vi "3.1.1_ECO_Power_Tune.vi"(6 "Data in":T1, 8 "error in (no error)":errorcluster, 9 "AllControls In":T2, 10 "?":T3, 11 "Message Queue out":T4) -> (0 "error out":errorcluster, 1 "Flow":string, 2 "Data":T3, 3 "Message Queue Out":T4, 4 "Data out":T1)   [LabVIEW 2017]
uses:
  Depends/AMC/subVIs/TypeDefs/amc_Message Queue.ctl
  Depends/AMC/subVIs/TypeDefs/amc_Message.ctl
  Depends/Tools/Keyed Array/Tools_KeyedArray KeyedArray.ctl
  Ctrls/Data.ctl
  Ctrls/CSV_Data.ctl
  Ctrls/AllControls.ctl
  DIPC 692 Daemon API/typdef/get_parameter.ctl
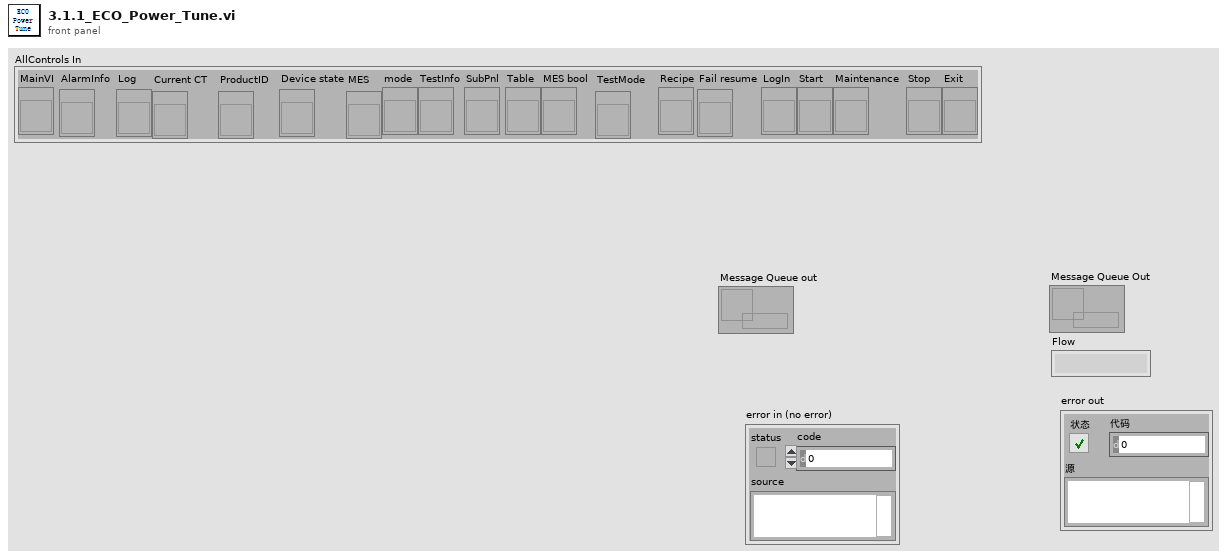
[diagram p1: front panel]
types:
  T1 = typedef "CSV_Data.ctl" = cluster{"Initialisation":cluster{"LMT - Connect UUT (con COM)":string, "LMT - Software Version (rrel)":string, "LMT - Write SKU file (wskuc)":string, "LMT - SKU file name":string, "Connect UUT DDM":string, "Read DDM EOL Timestamp - Mode":string, "Read DDM EOL Timestamp - Timestamp":string, "Read DDM EOL Timestamp - Rig ID":string, "Read DDM EOL Timestamp - Passmark ID":string, "Read DDM EOL Timestamp - Passmark Rev":string, "Software Version before flashing":string, "Read Hardware Serial":string, "UUT DDM SN":string, "Compare DDM SN with MES SN":string, "Backup PCBA Calibration EEPROM Response - CAL":string, "Flash Firmware Version":string, "Check SW Version":string, "Read DDM SW Version after flashing":string, "Set SKU Config":string, "Ready Status":string, "Set Device Mode to EOL":string, "DDM Parameter - Voltage":string, "DDM Parameter - Current":string, "DDM Parameter - Power":string, "DDM Parameter - Speed":string, "DDM Parameter - Pressure":string, "Tester Parameter - Voltage":string, "Tester Parameter - Current":string, "Tester Parameter - Power":string, "Tester Parameter - Ambient Pressure":string, "Tester Parameter - Ambient Temperature":string, "Calculated Parameter - DDM Pressure Corrected":string, "Calculated Parameter - DDM Real Power":string, "Calculated Parameter - Delta V":string}, "BEMF_Calibration":cluster{"Calibration Result - eol_cold_bemf_temp":string, "DDM Ambient Temp":string, "Restriction Plate Diameter":string, "Calibration Result - eol_bemf_mp_cold_coef_a":string, "Calibration Result - eol_bemf_mp_cold_coef_b":string, "Calibration Result - eol_bemf_mp_cold_coef_c":string, "Calibration Result - eol_bemf_lsi_cold_ref_coeffs":string, "Get - Calibration Result - eol_bemf_lsi_speed":string, "Get - Calibration Result - eol_bemf_lsi_integral_0":string, "Calibration Result - eol_bemf_lsi_integral_1":string, "Get - Calibration Result - eol_bemf_lsi_integral_2":string, "Get - Calibration Result - eol_cold_bemf":string, "Get - Calibration Result - eol_cold_bemf_fisf":string, "Finalise Calibration":string, "Compare -Calibration Result - eol_cold_bemf":string, "Compare -Calibration Result - eol_cold_bemf_fisf":string}, "ECO":cluster{"Reset Power Tune":string, "Reset BEMF FISF Calibration":string, "Restriction Plate Diameter":string, "ECO - Stabilisation Time":string, "ECO - DDM Parameter - Voltage":string, "ECO - DDM Parameter - Current":string, "ECO - DDM Parameter - Power":string, "ECO - DDM Parameter - Measured Power":string, "ECO - DDM Parameter - Speed":string, "ECO - DDM Parameter - Pressure":string, "ECO - Tester Parameter - Voltage":string, "ECO - Tester Parameter - Current":string, "ECO - Tester Parameter - Power":string, "ECO - Tester Parameter - Ambient Pressure":string, "ECO - Tester Parameter - Ambient Temperature":string, "ECO - Tester Parameter - Ambient Humidity":string, "ECO - Calculated Parameter - DDM Pressure Corrected":string, "ECO - Calculated Parameter - DDM Real Power":string, "ECO - Calculated Parameter - Delta V":string, "ECO - Calculated Parameter - Flowrate":string, "ECO - Calculated Parameter - Airwatt":string, "ECO - Formula":string, "PT ECO - Power Tune Mode Status":string}, "BOOST":cluster{"Restriction Plate Diameter":string, "BOOST - Stabilisation Time":string, "BOOST - DDM Parameter - Voltage":string, "BOOST - DDM Parameter - Current":string, "BOOST - DDM Parameter - Power":string, "BOOST - DDM Parameter - Measured Power":string, "BOOST - DDM Parameter - Speed":string, "BOOST - DDM Parameter - Pressure":string, "BOOST - Tester Parameter - Voltage":string, "BOOST - Tester Parameter - Current":string, "BOOST - Tester Parameter - Power":string, "BOOST - Tester Parameter - Ambient Pressure":string, "BOOST - Tester Parameter - Ambient Temperature":string, "BOOST - Tester Parameter - Ambient Humidity":string, "BOOST - Calculated Parameter - DDM Pressure Corrected":string, "BOOST - Calculated Parameter - DDM Real Power":string, "BOOST - Calculated Parameter - Delta V":string, "BOOST - Calculated Parameter - Flowrate":string, "BOOST - Calculated Parameter - Airwatt":string, "BOOST - Get AM Presence":string, "Air Muscle Turn Off Status":string, "BOOST - Air Muscle Calculated Parameter - Airwatt B":string, "BOOST - Air Muscle Calculate Airwatt Delta":string, "PT BOOST - Power Tune Mode Status":string, "Finalise Calibration":string, "ECO - Get AW Calibration value":string, "BOOST - Get AW Calibration value":string}, "MAX":cluster{"Restriction Plate Diameter":string, "MAX - Stabilisation Time":string, "Get Average Delta Tmag (LSIdelta_FISFdelta_LSItmag_FISFtmag_IIRtmag)":string, "Get Average Delta Tmag FISF":string, "MAX - DDM Parameter - Voltage":string, "MAX - DDM Parameter - Current":string, "MAX - DDM Parameter - Power":string, "MAX - DDM Parameter - Measured Power":string, "MAX - DDM Parameter - Speed":string, "MAX - DDM Parameter - Pressure":string, "MAX - Tester Parameter - Voltage":string, "MAX - Tester Parameter - Current":string, "MAX - Tester Parameter - Power":string, "MAX - Tester Parameter - Ambient Pressure":string, "MAX - Tester Parameter - Ambient Temperature":string, "MAX - Tester Parameter - Ambient Humidity":string, "MAX - Calculated Parameter - DDM Pressure Corrected":string, "MAX - Calculated Parameter - DDM Real Power":string, "MAX - Calculated Parameter - Delta V":string, "MAX - Calculated Parameter - Flowrate":string, "MAX - Calculated Parameter - Airwatt":string, "MAX_FISF_Check_Average_Delta_Tmag":string, "MAX - FISF - BEMF Finetune Result":string, "MAX tune - Delta P1":string, "MAX tune - Calculated Parameter - Airwatt":string, "Calculate Delta Airwatts - MAX finetune - Delta P2":string, "MAX finetune - DDM Parameter - Voltage":string, "MAX finetune - DDM Parameter - Current":string, "MAX finetune - DDM Parameter - Power":string, "MAX finetune - DDM Parameter - Measured Power":string, "MAX finetune - DDM Parameter - Speed":string, "MAX finetune - DDM Parameter - Pressure":string, "MAX finetune - Tester Parameter - Voltage":string, "MAX finetune - Tester Parameter - Current":string, "MAX finetune - Tester Parameter - Power":string, "MAX finetune - Tester Parameter - Ambient Pressure":string, "MAX finetune - Tester Parameter - Ambient Temperature":string, "MAX finetune - Tester Parameter - Ambient Humidity":string, "MAX finetune - Calculated Parameter - DDM Pressure Corrected":string, "MAX finetune - Calculated Parameter - DDM Real Power":string, "MAX finetune - Calculated Parameter - Delta V":string, "MAX finetune - Calculated Parameter - Flowrate":string, "MAX finetune - Calculated Parameter - Airwatt":string, "Check Derate Result":string, "Delta Tmag FISF":string, "Get Hot BEMF Result":string, "Calculate delta Pressure":string, "Finalise Calibration":string, "Calculate & Check Delta BEMF":string, "Delta P Airwatts Value":string}, "LL":cluster{"DDM Ambient Temp":string, "Restriction Plate Diameter":string, "LL - DDM Parameter - Voltage":string, "LL - DDM Parameter - Current":string, "LL - DDM Parameter - Power":string, "LL - DDM Parameter - Measured Power":string, "LL - DDM Parameter - Speed":string, "LL - DDM Parameter - Pressure":string, "LL - Tester Parameter - Voltage":string, "LL - Tester Parameter - Current":string, "LL - Tester Parameter - Power":string, "LL - DDM Real Power":string, "LL - Calibrate Task Detect LL":string}, "HL":cluster{"HL - DDM Parameter - Voltage":string, "HL - DDM Parameter - Current":string, "HL - DDM Parameter - Power":string, "HL - DDM Parameter - Measured Power":string, "HL - DDM Parameter - Speed":string, "HL - DDM Parameter - Pressure":string, "HL - Tester Parameter - Voltage":string, "HL - Tester Parameter - Current":string, "HL - Tester Parameter - Power":string, "HL - DDM Real Power":string, "HL - Calibrate Task Detect HL":string}, "LH":cluster{"Restriction Plate Diameter":string, "LH - DDM Parameter - Voltage":string, "LH - DDM Parameter - Current":string, "LH - DDM Parameter - Power":string, "LH - DDM Parameter - Measured Power":string, "LH - DDM Parameter - Speed":string, "LH - DDM Parameter - Pressure":string, "LH - Tester Parameter - Voltage":string, "LH - Tester Parameter - Current":string, "LH - Tester Parameter - Power":string, "LH - DDM Real Power":string, "LH - Calibrate Task Detect LH":string}, "HH":cluster{"HH - DDM Parameter - Voltage":string, "HH - DDM Parameter - Current":string, "HH - DDM Parameter - Power":string, "HH - DDM Parameter - Measured Power":string, "HH - DDM Parameter - Speed":string, "HH - DDM Parameter - Pressure":string, "HH - Tester Parameter - Voltage":string, "HH - Tester Parameter - Current":string, "HH - Tester Parameter - Power":string, "HH - DDM Real Power":string, "HH - Calibrate Task Detect HH":string}, "Inlet Blockage Calibration":cluster{"Inlet Blockage Calibration - DDM Parameter - Voltage":string, "Inlet Blockage Calibration - DDM Parameter - Current":string, "Inlet Blockage Calibration - DDM Parameter - Power":string, "Inlet Blockage Calibration - DDM Parameter - Measured Power":string, "Inlet Blockage Calibration - DDM Parameter - Speed":string, "Inlet Blockage Calibration - DDM Parameter - Pressure":string, "Inlet Blockage Calibration - Tester Parameter - Voltage":string, "Inlet Blockage Calibration - Tester Parameter - Current":string, "Inlet Blockage Calibration - Tester Parameter - Power":string, "Inlet Blockage Calibration - DDM Real Power":string, "Calibration Inlet Blockage_E":string, "Finalise Calibration":string, "Get Task Detect LL":string, "Get Task Detect HL":string, "Get Task Detect LH":string, "Get Task Detect HH":string, "Calibration Inlet Blockage":string, "Calibration eol cold bemf temp":string}, "GOOD":cluster{"GOOD UNIT - Clear EEPROM Error Log":string, "GOOD UNIT - Write Product Timestamp - Mode":string, "GOOD UNIT - Write Product Timestamp - Timestamp":string, "GOOD UNIT - Write Product Timestamp - Rig ID":string, "GOOD UNIT - Write Product Timestamp - Passmark ID":string, "GOOD UNIT - Write Product Timestamp - Passmark Rev":string, "GOOD UNIT - Set Device Mode to PROD":string, "GOOD UNIT - Backup PCBA Calibration EEPROM Response":string, "GOOD UNIT - Check Security Bit":string, "GOOD UNIT - Set Calibration Lock":string, "GOOD UNIT - Get_Calibration_Lock":string, "GOOD UNIT - Disconnect UUT":string}, "NG":cluster{"NG UNIT - Read NVM Error":string, "NG UNIT - Set Device Mode to FCT":string, "NG UNIT - Backup PCBA Calibration EEPROM Response - CAL":string, "NG UNIT - Backup PCBA Calibration EEPROM Response - ERROR":string, "NG UNIT - Backup PCBA Calibration EEPROM Response - USAGE":string, "NG UNIT - Disconnect UUT":string}, "SN":string, "Table":string[][], "Count":cluster{"Total":i32, "OK":i32, "NG":i32, "Yield":dbl}, "Start Time":timestamp, "daemon reference":refnum<k5>, "CT":dbl, "Config":string[][], "OK/NG":bool, "Station ID":string, "MES DDM SN":string, "MES PCBA SN":string, "Retest":string, "Lux":string, "Initialisation_Status":cluster{"LMT - Connect UUT (con COM)":string, "LMT - Software Version (rrel)":string, "LMT - Write SKU file (wskuc)":string, "LMT - SKU file name":string, "Connect UUT DDM":string, "Read DDM EOL Timestamp - Mode":string, "Read DDM EOL Timestamp - Timestamp":string, "Read DDM EOL Timestamp - Rig ID":string, "Read DDM EOL Timestamp - Passmark ID":string, "Read DDM EOL Timestamp - Passmark Rev":string, "Software Version before flashing":string, "Read Hardware Serial":string, "UUT DDM SN":string, "Compare DDM SN with MES SN":string, "Backup PCBA Calibration EEPROM Response - CAL":string, "Flash Firmware Version":string, "Check SW Version":string, "Read DDM SW Version after flashing":string, "Set SKU Config":string, "Ready Status":string, "Set Device Mode to EOL":string, "DDM Parameter - Voltage":string, "DDM Parameter - Current":string, "DDM Parameter - Power":string, "DDM Parameter - Speed":string, "DDM Parameter - Pressure":string, "Tester Parameter - Voltage":string, "Tester Parameter - Current":string, "Tester Parameter - Power":string, "Tester Parameter - Ambient Pressure":string, "Tester Parameter - Ambient Temperature":string, "Calculated Parameter - DDM Pressure Corrected":string, "Calculated Parameter - DDM Real Power":string, "Calculated Parameter - Delta V":string}, "BEMF_Calibration_Status":cluster{"Calibration Result - eol_cold_bemf_temp":string, "DDM Ambient Temp":string, "Restriction Plate Diameter":string, "Calibration Result - eol_bemf_mp_cold_coef_a":string, "Calibration Result - eol_bemf_mp_cold_coef_b":string, "Calibration Result - eol_bemf_mp_cold_coef_c":string, "Calibration Result - eol_bemf_lsi_cold_ref_coeffs":string, "Get - Calibration Result - eol_bemf_lsi_speed":string, "Get - Calibration Result - eol_bemf_lsi_integral_0":string, "Calibration Result - eol_bemf_lsi_integral_1":string, "Get - Calibration Result - eol_bemf_lsi_integral_2":string, "Get - Calibration Result - eol_cold_bemf":string, "Get - Calibration Result - eol_cold_bemf_fisf":string, "Finalise Calibration":string, "Compare -Calibration Result - eol_cold_bemf":string, "Compare -Calibration Result - eol_cold_bemf_fisf":string}, "ECO_Status":cluster{"Reset Power Tune":string, "Reset BEMF FISF Calibration":string, "Restriction Plate Diameter":string, "ECO - Stabilisation Time":string, "ECO - DDM Parameter - Voltage":string, "ECO - DDM Parameter - Current":string, "ECO - DDM Parameter - Power":string, "ECO - DDM Parameter - Measured Power":string, "ECO - DDM Parameter - Speed":string, "ECO - DDM Parameter - Pressure":string, "ECO - Tester Parameter - Voltage":string, "ECO - Tester Parameter - Current":string, "ECO - Tester Parameter - Power":string, "ECO - Tester Parameter - Ambient Pressure":string, "ECO - Tester Parameter - Ambient Temperature":string, "ECO - Tester Parameter - Ambient Humidity":string, "ECO - Calculated Parameter - DDM Pressure Corrected":string, "ECO - Calculated Parameter - DDM Real Power":string, "ECO - Calculated Parameter - Delta V":string, "ECO - Calculated Parameter - Flowrate":string, "ECO - Calculated Parameter - Airwatt":string, "ECO - Formula":string, "PT ECO - Power Tune Mode Status":string}, "BOOST_Status":cluster{"Restriction Plate Diameter":string, "BOOST - Stabilisation Time":string, "BOOST - DDM Parameter - Voltage":string, "BOOST - DDM Parameter - Current":string, "BOOST - DDM Parameter - Power":string, "BOOST - DDM Parameter - Measured Power":string, "BOOST - DDM Parameter - Speed":string, "BOOST - DDM Parameter - Pressure":string, "BOOST - Tester Parameter - Voltage":string, "BOOST - Tester Parameter - Current":string, "BOOST - Tester Parameter - Power":string, "BOOST - Tester Parameter - Ambient Pressure":string, "BOOST - Tester Parameter - Ambient Temperature":string, "BOOST - Tester Parameter - Ambient Humidity":string, "BOOST - Calculated Parameter - DDM Pressure Corrected":string, "BOOST - Calculated Parameter - DDM Real Power":string, "BOOST - Calculated Parameter - Delta V":string, "BOOST - Calculated Parameter - Flowrate":string, "BOOST - Calculated Parameter - Airwatt":string, "BOOST - Get AM Presence":string, "Air Muscle Turn Off Status":string, "BOOST - Air Muscle Calculated Parameter - Airwatt B":string, "BOOST - Air Muscle Calculate Airwatt Delta":string, "PT BOOST - Power Tune Mode Status":string, "Finalise Calibration":string, "ECO - Get AW Calibration value":string, "BOOST - Get AW Calibration value":string}, "MAX_Status":cluster{"Restriction Plate Diameter":string, "MAX - Stabilisation Time":string, "Get Average Delta Tmag (LSIdelta_FISFdelta_LSItmag_FISFtmag_IIRtmag)":string, "Get Average Delta Tmag FISF":string, "MAX - DDM Parameter - Voltage":string, "MAX - DDM Parameter - Current":string, "MAX - DDM Parameter - Power":string, "MAX - DDM Parameter - Measured Power":string, "MAX - DDM Parameter - Speed":string, "MAX - DDM Parameter - Pressure":string, "MAX - Tester Parameter - Voltage":string, "MAX - Tester Parameter - Current":string, "MAX - Tester Parameter - Power":string, "MAX - Tester Parameter - Ambient Pressure":string, "MAX - Tester Parameter - Ambient Temperature":string, "MAX - Tester Parameter - Ambient Humidity":string, "MAX - Calculated Parameter - DDM Pressure Corrected":string, "MAX - Calculated Parameter - DDM Real Power":string, "MAX - Calculated Parameter - Delta V":string, "MAX - Calculated Parameter - Flowrate":string, "MAX - Calculated Parameter - Airwatt":string, "MAX_FISF_Check_Average_Delta_Tmag":string, "MAX - FISF - BEMF Finetune Result":string, "MAX tune - Delta P1":string, "MAX tune - Calculated Parameter - Airwatt":string, "Calculate Delta Airwatts - MAX finetune - Delta P2":string, "MAX finetune - DDM Parameter - Voltage":string, "MAX finetune - DDM Parameter - Current":string, "MAX finetune - DDM Parameter - Power":string, "MAX finetune - DDM Parameter - Measured Power":string, "MAX finetune - DDM Parameter - Speed":string, "MAX finetune - DDM Parameter - Pressure":string, "MAX finetune - Tester Parameter - Voltage":string, "MAX finetune - Tester Parameter - Current":string, "MAX finetune - Tester Parameter - Power":string, "MAX finetune - Tester Parameter - Ambient Pressure":string, "MAX finetune - Tester Parameter - Ambient Temperature":string, "MAX finetune - Tester Parameter - Ambient Humidity":string, "MAX finetune - Calculated Parameter - DDM Pressure Corrected":string, "MAX finetune - Calculated Parameter - DDM Real Power":string, "MAX finetune - Calculated Parameter - Delta V":string, "MAX finetune - Calculated Parameter - Flowrate":string, "MAX finetune - Calculated Parameter - Airwatt":string, "Check Derate Result":string, "Delta Tmag FISF":string, "Get Hot BEMF Result":string, "Calculate delta Pressure":string, "Finalise Calibration":string, "Calculate & Check Delta BEMF":string, "Delta P Airwatts Value":string}, "LL_Status":cluster{"DDM Ambient Temp":string, "Restriction Plate Diameter":string, "LL - DDM Parameter - Voltage":string, "LL - DDM Parameter - Current":string, "LL - DDM Parameter - Power":string, "LL - DDM Parameter - Measured Power":string, "LL - DDM Parameter - Speed":string, "LL - DDM Parameter - Pressure":string, "LL - Tester Parameter - Voltage":string, "LL - Tester Parameter - Current":string, "LL - Tester Parameter - Power":string, "LL - DDM Real Power":string, "LL - Calibrate Task Detect LL":string}, "HL_Status":cluster{"HL - DDM Parameter - Voltage":string, "HL - DDM Parameter - Current":string, "HL - DDM Parameter - Power":string, "HL - DDM Parameter - Measured Power":string, "HL - DDM Parameter - Speed":string, "HL - DDM Parameter - Pressure":string, "HL - Tester Parameter - Voltage":string, "HL - Tester Parameter - Current":string, "HL - Tester Parameter - Power":string, "HL - DDM Real Power":string, "HL - Calibrate Task Detect HL":string}, "LH_Status":cluster{"Restriction Plate Diameter":string, "LH - DDM Parameter - Voltage":string, "LH - DDM Parameter - Current":string, "LH - DDM Parameter - Power":string, "LH - DDM Parameter - Measured Power":string, "LH - DDM Parameter - Speed":string, "LH - DDM Parameter - Pressure":string, "LH - Tester Parameter - Voltage":string, "LH - Tester Parameter - Current":string, "LH - Tester Parameter - Power":string, "LH - DDM Real Power":string, "LH - Calibrate Task Detect LH":string}, "HH_Status":cluster{"HH - DDM Parameter - Voltage":string, "HH - DDM Parameter - Current":string, "HH - DDM Parameter - Power":string, "HH - DDM Parameter - Measured Power":string, "HH - DDM Parameter - Speed":string, "HH - DDM Parameter - Pressure":string, "HH - Tester Parameter - Voltage":string, "HH - Tester Parameter - Current":string, "HH - Tester Parameter - Power":string, "HH - DDM Real Power":string, "HH - Calibrate Task Detect HH":string}, "Inlet Blockage Calibration_Status":cluster{"Inlet Blockage Calibration - DDM Parameter - Voltage":string, "Inlet Blockage Calibration - DDM Parameter - Current":string, "Inlet Blockage Calibration - DDM Parameter - Power":string, "Inlet Blockage Calibration - DDM Parameter - Measured Power":string, "Inlet Blockage Calibration - DDM Parameter - Speed":string, "Inlet Blockage Calibration - DDM Parameter - Pressure":string, "Inlet Blockage Calibration - Tester Parameter - Voltage":string, "Inlet Blockage Calibration - Tester Parameter - Current":string, "Inlet Blockage Calibration - Tester Parameter - Power":string, "Inlet Blockage Calibration - DDM Real Power":string, "Calibration Inlet Blockage_E":string, "Finalise Calibration":string, "Get Task Detect LL":string, "Get Task Detect HL":string, "Get Task Detect LH":string, "Get Task Detect HH":string, "Calibration Inlet Blockage":string, "Calibration eol cold bemf temp":string}, "GOOD_Status":cluster{"GOOD UNIT - Clear EEPROM Error Log":string, "GOOD UNIT - Write Product Timestamp - Mode":string, "GOOD UNIT - Write Product Timestamp - Timestamp":string, "GOOD UNIT - Write Product Timestamp - Rig ID":string, "GOOD UNIT - Write Product Timestamp - Passmark ID":string, "GOOD UNIT - Write Product Timestamp - Passmark Rev":string, "GOOD UNIT - Set Device Mode to PROD":string, "GOOD UNIT - Backup PCBA Calibration EEPROM Response":string, "GOOD UNIT - Check Security Bit":string, "GOOD UNIT - Set Calibration Lock":string, "GOOD UNIT - Get_Calibration_Lock":string, "GOOD UNIT - Disconnect UUT":string}, "NG_Status":cluster{"NG UNIT - Read NVM Error":string, "NG UNIT - Set Device Mode to FCT":string, "NG UNIT - Backup PCBA Calibration EEPROM Response - CAL":string, "NG UNIT - Backup PCBA Calibration EEPROM Response - ERROR":string, "NG UNIT - Backup PCBA Calibration EEPROM Response - USAGE":string, "NG UNIT - Disconnect UUT":string}, "SKU":string, "Plate_Diameter":string, "Alarm":string}
  T2 = typedef "AllControls.ctl" = cluster{"MainVI":refnum<vi>, "AlarmInfo":refnum<vi>, "Log":refnum<vi>, "Current CT":refnum<vi>, "ProductID":refnum<vi>, "Device state":refnum<vi>, "MES":refnum<vi>, "mode":refnum<vi>, "TestInfo":refnum<vi>, "SubPnl":refnum<vi>, "Table":refnum<vi>, "MES bool":refnum<vi>, "TestMode":refnum<vi>, "Recipe":refnum<vi>, "Fail resume":refnum<vi>, "LogIn":refnum<vi>, "Start":refnum<vi>, "Maintenance":refnum<vi>, "Stop":refnum<vi>, "Exit":refnum<vi>}
  T3 = typedef "Data.ctl" = cluster{"Initialisation":cluster{"DDM_Parameter":dbl[], "DDM_Parameter_status":bool[], "Get_Tester_Parameter":dbl[], "Get_Tester_Parameter_status":bool[], "Cal_Tester_Parameter":dbl[], "Cal_Tester_Parameter_status":bool[], "sw_version_before_status":bool, "sw_version_after_status":bool, "Set_SKU_Config_With_LMT_status":bool, "FCT_timestamp_status":bool, "LMT_Connect_to_UUT_status":bool}, "BEMF_Calibration":cluster{"Read_ambient_temperature":dbl, "Calibration_Vaule":dbl[], "Calibration_Vaule _B":dbl[], "Calibration_Vaule_status":bool[], "Calibration_Vaule_B_status":bool[]}, "ECO":cluster{"DDM_Parameter":dbl[], "DDM_Parameter_status":bool[], "Get_Tester_Parameter":dbl[], "Get_Tester_Parameter_status":bool[], "Cal_Tester_Parameter":dbl[], "Cal_Tester_Parameter_status":bool[], "DDM_Parameter_after_power_tune":dbl[], "Get_Tester_Parameter_after_power_tune":dbl[], "Cal_Tester_Parameter_after_power_tune":dbl[], "Cal_Tester_Parameter_after_power_tune_status":bool[], "Delta_P":dbl}, "BOOST":cluster{"DDM_Parameter":dbl[], "DDM_Parameter_status":bool[], "Get_Tester_Parameter":dbl[], "Get_Tester_Parameter_status":bool[], "Cal_Tester_Parameter":dbl[], "Cal_Tester_Parameter_status":bool[], "DDM_Parameter_after_power_tune":dbl[], "Get_Tester_Parameter_after_power_tune":dbl[], "Cal_Tester_Parameter_after_power_tune":dbl[], "Cal_Tester_Parameter_after_power_tune_status":bool[], "airwatts_am_off":dbl, "AW_Delta_(AM_on_and_off)":dbl, "AW_Delta_(AM_on_and_off)_Status":bool, "Delta_P":dbl}, "MAX":cluster{"Average_Tmag_Data":cluster{"LSI Delta in degC":dbl, "FISF Delta in degc":dbl, "LSI Tmag in degC":dbl, "Fisf Tmag in degC":dbl, "IIR Tmag in degC":dbl}, "DDM_Parameter":dbl[], "DDM_Parameter_status":bool[], "Get_Tester_Parameter":dbl[], "Get_Tester_Parameter_status":bool[], "Cal_Tester_Parameter":dbl[], "BEMF_Finetune":cluster{"eol_bemf_mp_cold_coef_c":dbl, "eol_cold_bemf_fisf_offset":dbl}, "AW_Tune":cluster{"delta_P1":dbl, "delta_P_Setting":dbl}, "DDM_Parameter_after_Airwatts_Tune":dbl[], "Get_Tester_Parameter_after_Airwatts_Tune":dbl[], "Cal_Tester_Parameter_after_Airwatts_Tune":dbl[], "DDM_Parameter_after_Airwatts_Finetune":dbl[], "Get_Tester_Parameter_after_Airwatts_Finetune":dbl[], "Cal_Tester_Parameter_after_Airwatts_Finetune":dbl[], "AW_Finetune":cluster{"delta_P2":dbl, "delta_P_Setting":dbl}, "Delta_Tmag_after_tune":cluster{"LSI Delta in degC":dbl, "FISF Delta in degc":dbl, "LSI Tmag in degC":dbl, "Fisf Tmag in degC":dbl, "IIR Tmag in degC":dbl}, "Hot Bemf in mV":dbl, "DDM_Pressure":dbl, "Delta_Pressure":dbl, " Cold Bemf in mV":dbl, " delta Bemf":dbl, " delta p":dbl, "Delta_Pressure_status":bool, " delta Bemf_status":bool, "LSI Delta in degC_status":bool, "FISF Delta in degc_status":bool, "Max_check_derate_status_status":bool, "Average_All_data":dbl[][], "Average_Tmag_Data_status":bool[], "Average_Tmag_Data_after_tune_status":bool[], "Cal_Tester_Parameter_status":bool[], "Cal_Tester_Parameter_status_after_Airwatts_Tune":bool[], "Cal_Tester_Parameter_status_after_Airwatts_FineTune":bool[]}, "Task_Detect_Calib":cluster{"LL":cluster{"DDM_Parameter":dbl[], "DDM_Parameter_status":bool[], "Get_Tester_Parameter":dbl[], "Get_Tester_Parameter_status":bool[], "Set_task_detect_A":dbl, "Set_task_detect_A_Status":bool}, "HL":cluster{"DDM_Parameter":dbl[], "DDM_Parameter_status":bool[], "Get_Tester_Parameter":dbl[], "Get_Tester_Parameter_status":bool[], "Set_task_detect_B":dbl, "Set_task_detect_B_Status":bool}, "LH":cluster{"DDM_Parameter":dbl[], "DDM_Parameter_status":bool[], "Get_Tester_Parameter":dbl[], "Get_Tester_Parameter_status":bool[], "Set_task_detect_C":dbl, "Set_task_detect_C_Status":bool}, "HH":cluster{"DDM_Parameter":dbl[], "DDM_Parameter_status":bool[], "Get_Tester_Parameter":dbl[], "Get_Tester_Parameter_status":bool[], "Set_task_detect_D":dbl, "Read_and_check_calibration_Status":bool[], "Set_task_detect_D_Status":bool}, "Get_eol_inlet_blockage_E":dbl, "Calib_vaule":cluster{"Get_task_detect_LL":dbl, "Get_task_detect_HL":dbl, "Get_task_detect_LH":dbl, "Get_task_detect_HH":dbl, "eol_inlet_blockage":dbl, "eol_code_bemf_temp":dbl}, "calibrated temp":dbl, "Inlet_Blockage_Calibration":cluster{"DDM_Parameter":dbl[], "DDM_Parameter_status":bool[], "Get_Tester_Parameter":dbl[], "Get_Tester_Parameter_status":bool[]}, "Get_eol_inlet_blockage_E_Status":bool}, "good":cluster{"Write_Product_TS":cluster{"TIMESTAMP":i64, "RIG_ID":i64, "PASSMARK_ID":i64, "PASSMARK_REV":i64}, "Read_Product_TS":cluster{"TIMESTAMP":i64, "RIG_ID":i64, "PASSMARK_ID":i64, "PASSMARK_REV":i64}, "Good_Check_Secuity_Bit_Stauts":bool}}
  T4 = typedef "amc_Message Queue.ctl" = refnum<queue>
  T5 = typedef "HD Config.ctl" = cluster{" PC":cluster{"PC Address":u8[], "PC Port":i32}, "FCO":cluster{"COM":refnum<visa-resource-name>, "Baudrate":u32}, "DC Power ":cluster{"COM":refnum<visa-resource-name>, "Baudrate":u32}, "PW3336":cluster{"COM":refnum<visa-resource-name>, "Baudrate":u32}, "Lefoo":cluster{"COM":refnum<visa-resource-name>, "Baudrate":u32}, "Tempt&Hum":cluster{"COM":refnum<visa-resource-name>, "Baudrate":u32}, "DIPC":cluster{"COM":refnum<visa-resource-name>}, "Daemon":cluster{"IP Address":string, "Port":u16, "Retry":u16}, "NFC":cluster{"COM":refnum<visa-resource-name>, "Baudrate":u32}, "Fail_resume_mode":bool, "GRR":bool}
  T6 = typedef "get_parameter.ctl" = string
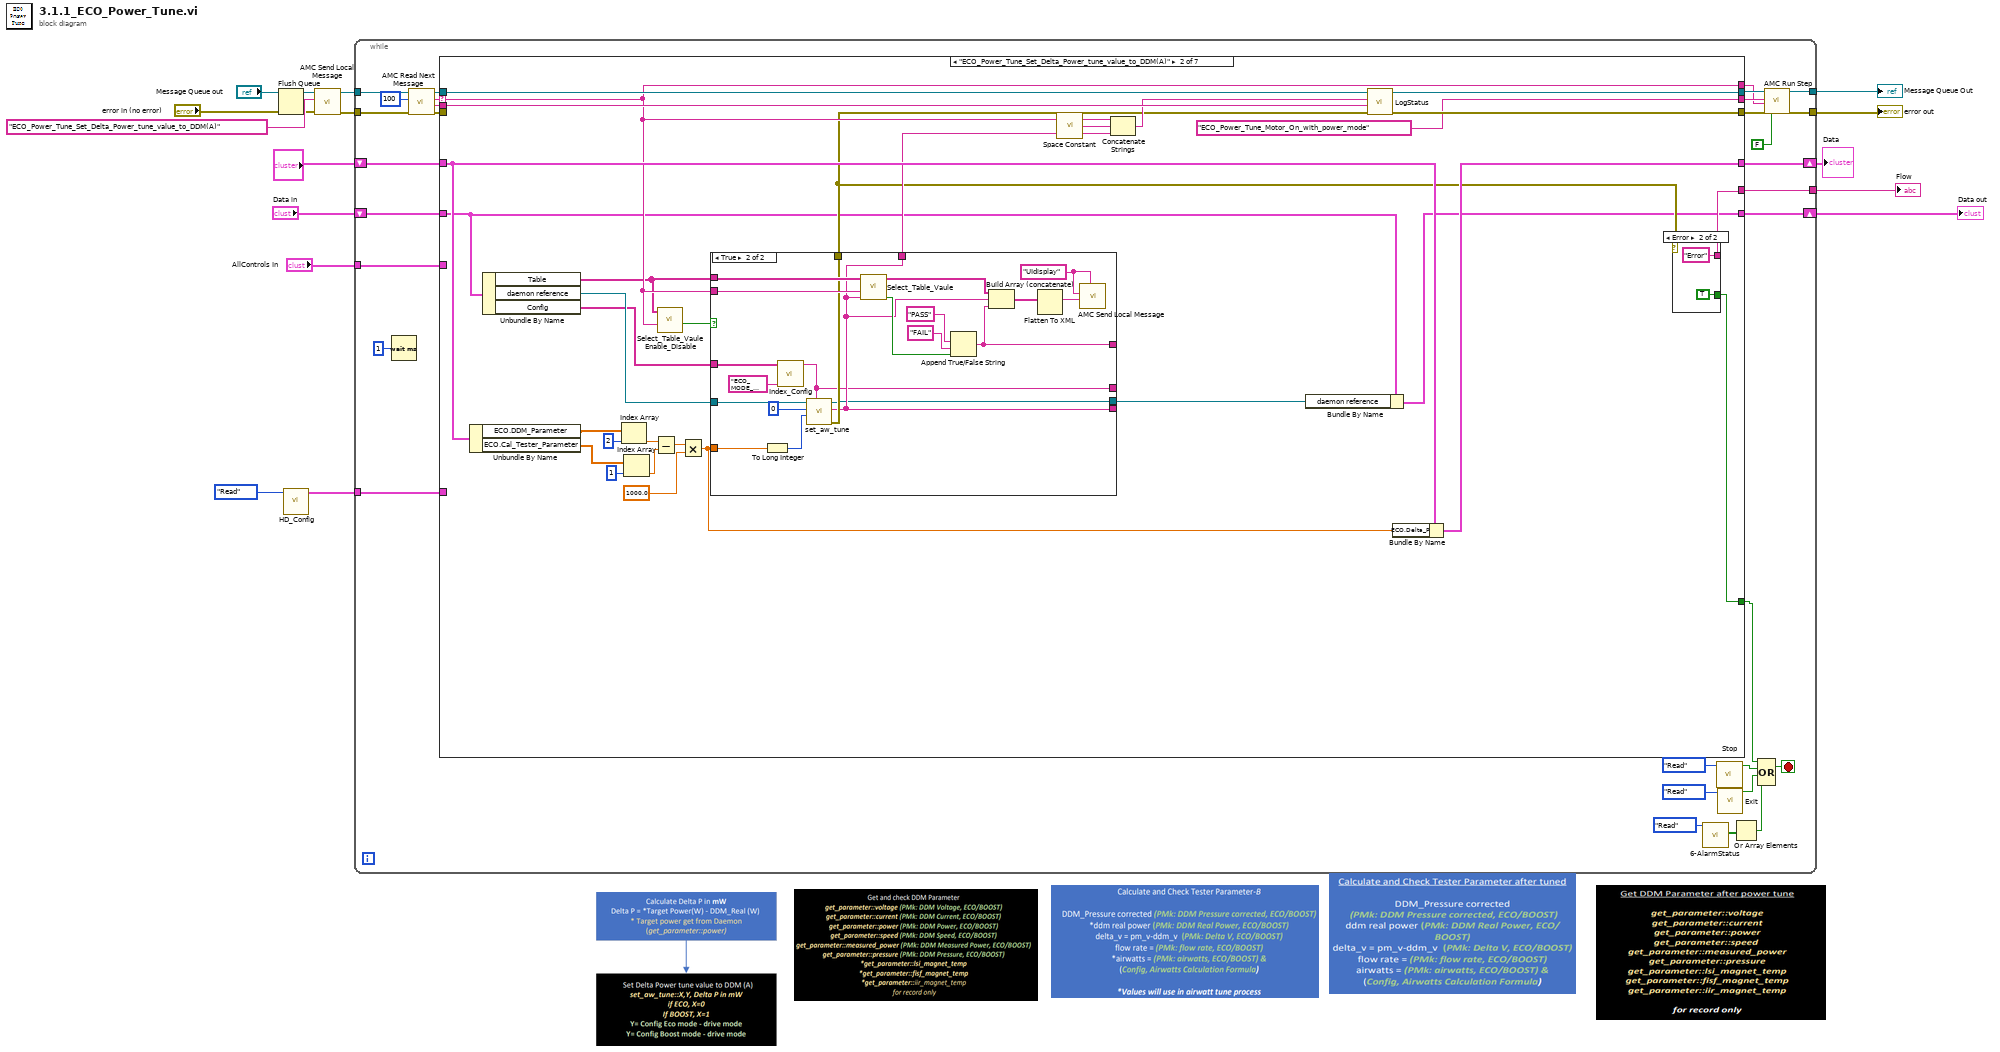
[diagram p0: block diagram]
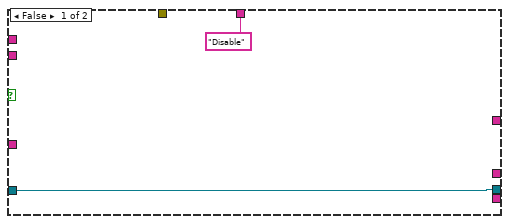
[diagram p4: hidden frame]
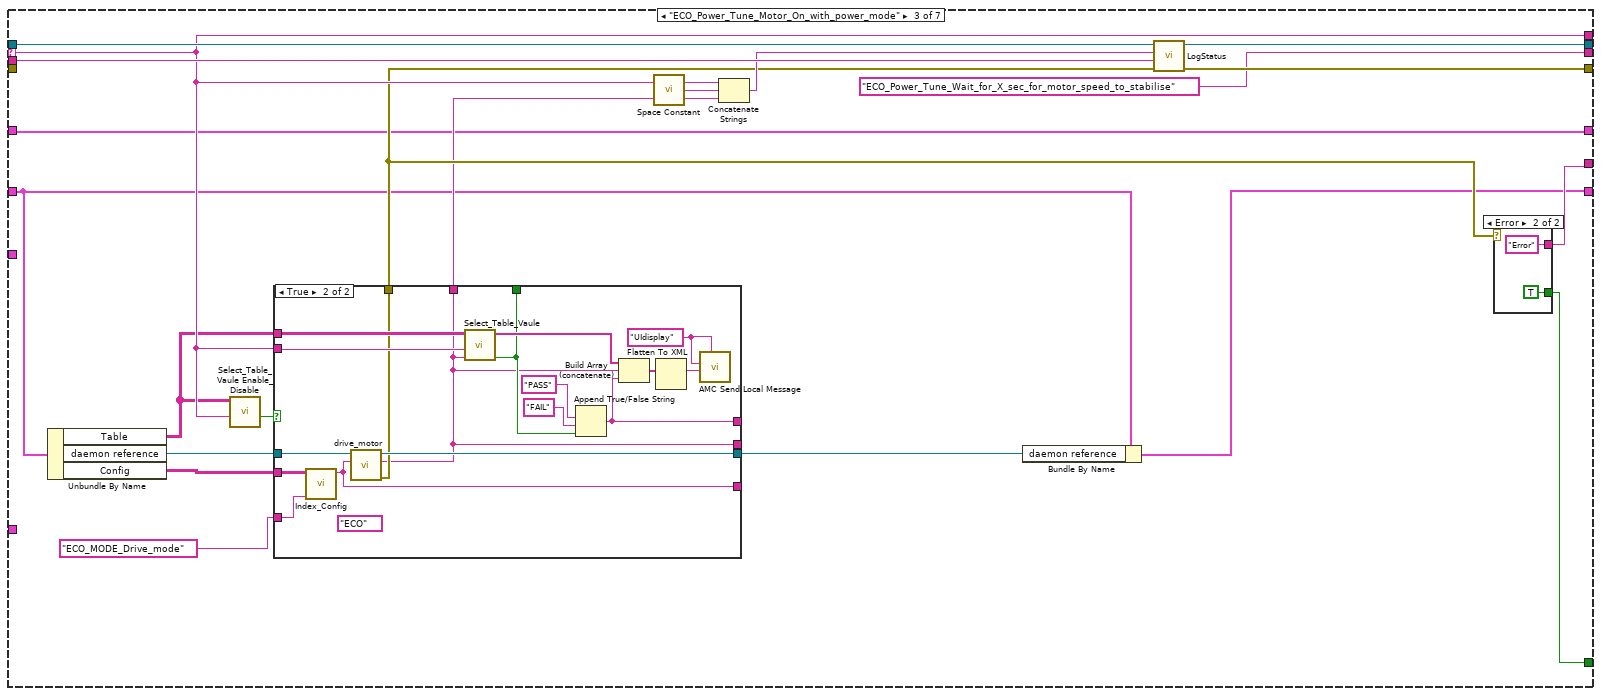
[diagram p5: hidden frame]
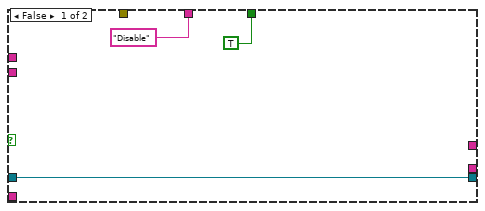
[diagram p7: hidden frame]
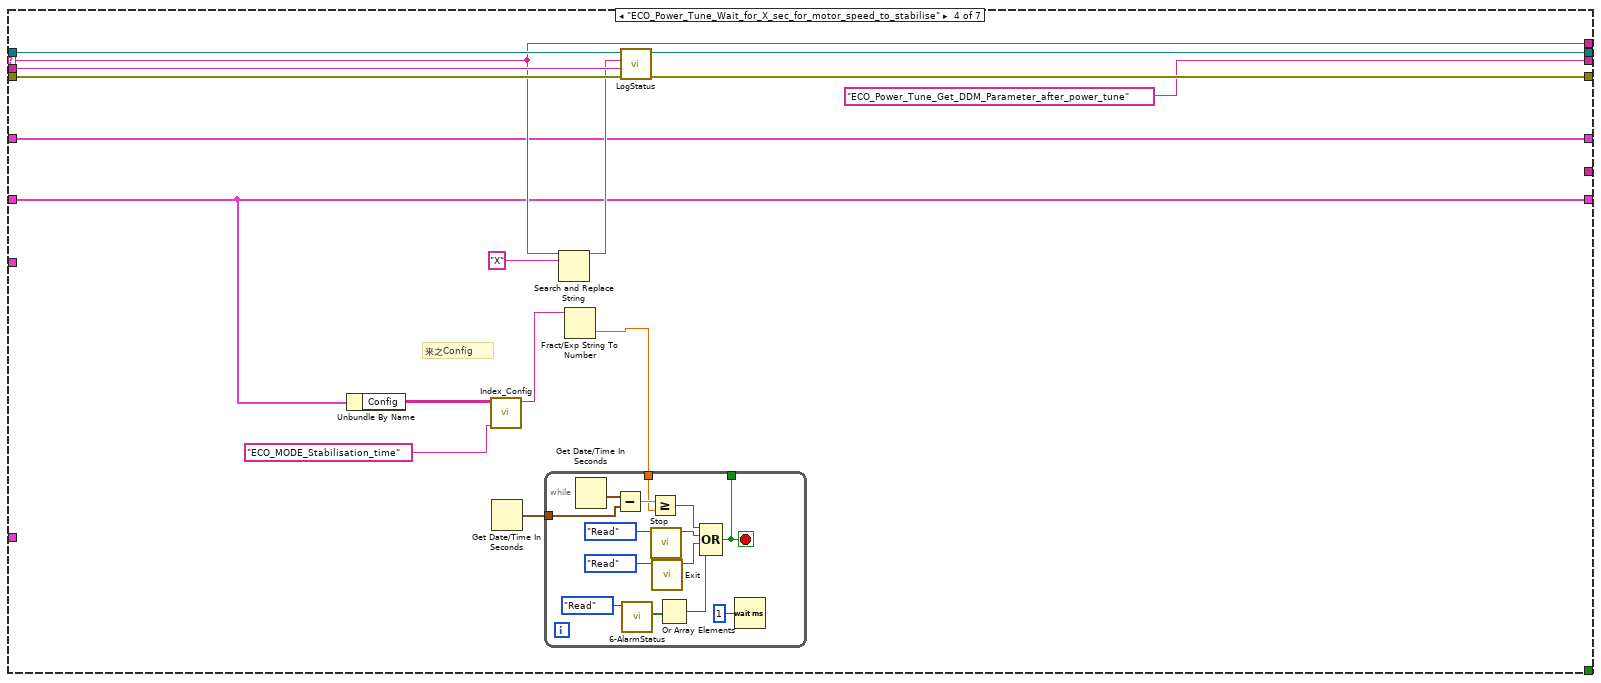
[diagram p8: hidden frame]
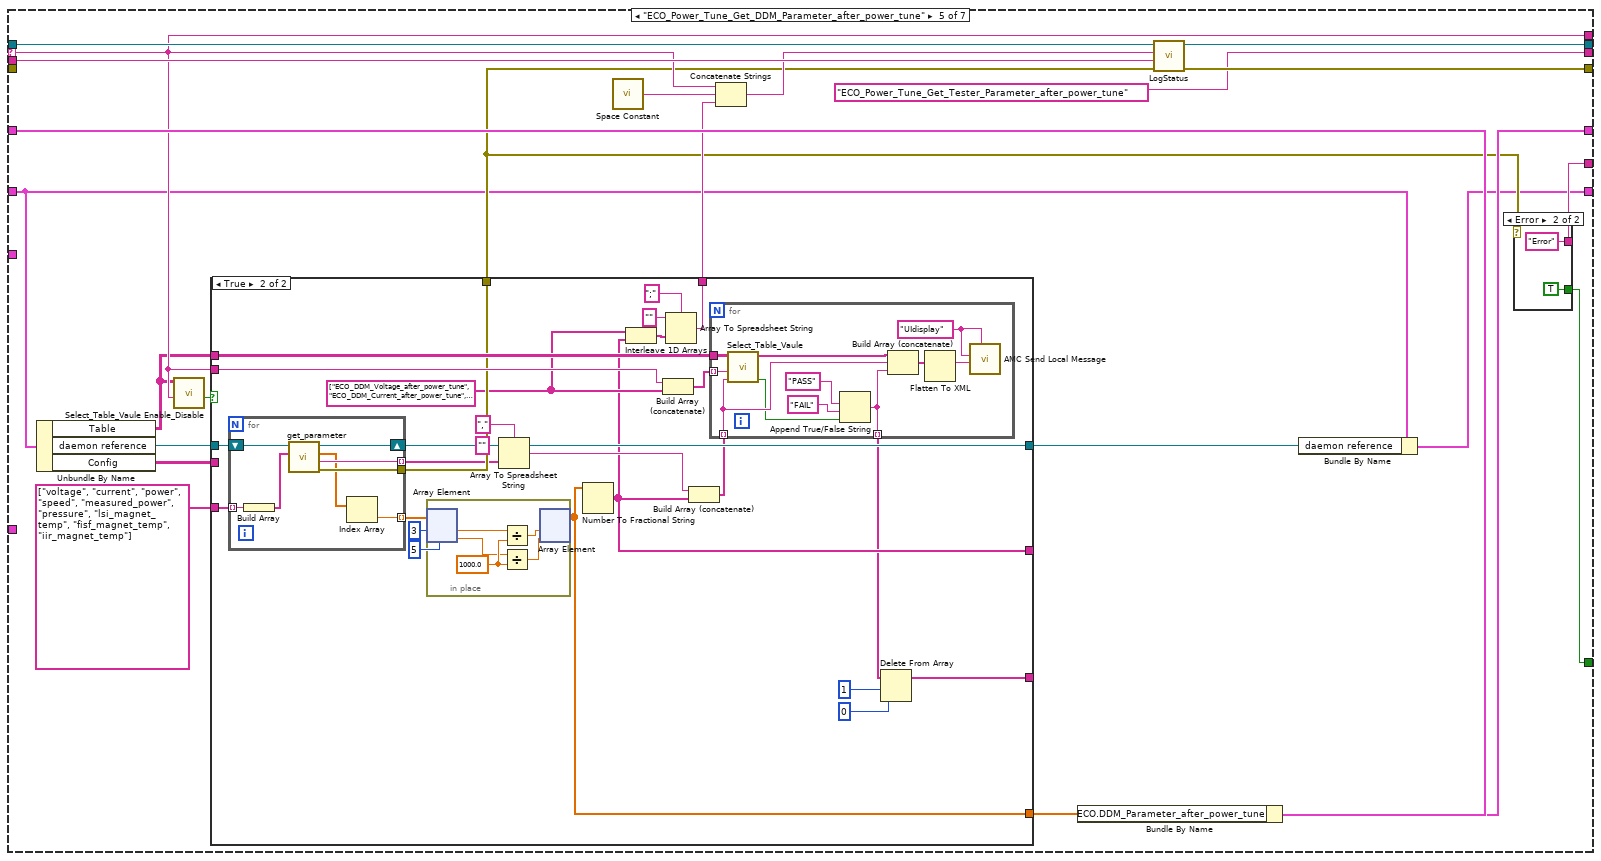
[diagram p9: hidden frame]
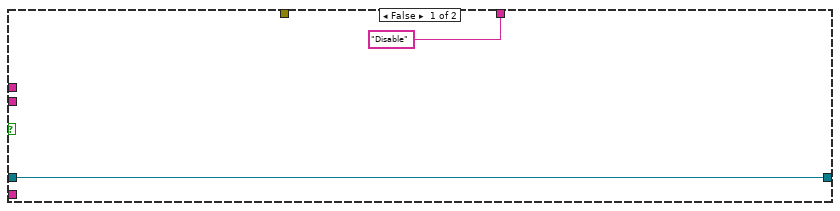
[diagram p11: hidden frame]
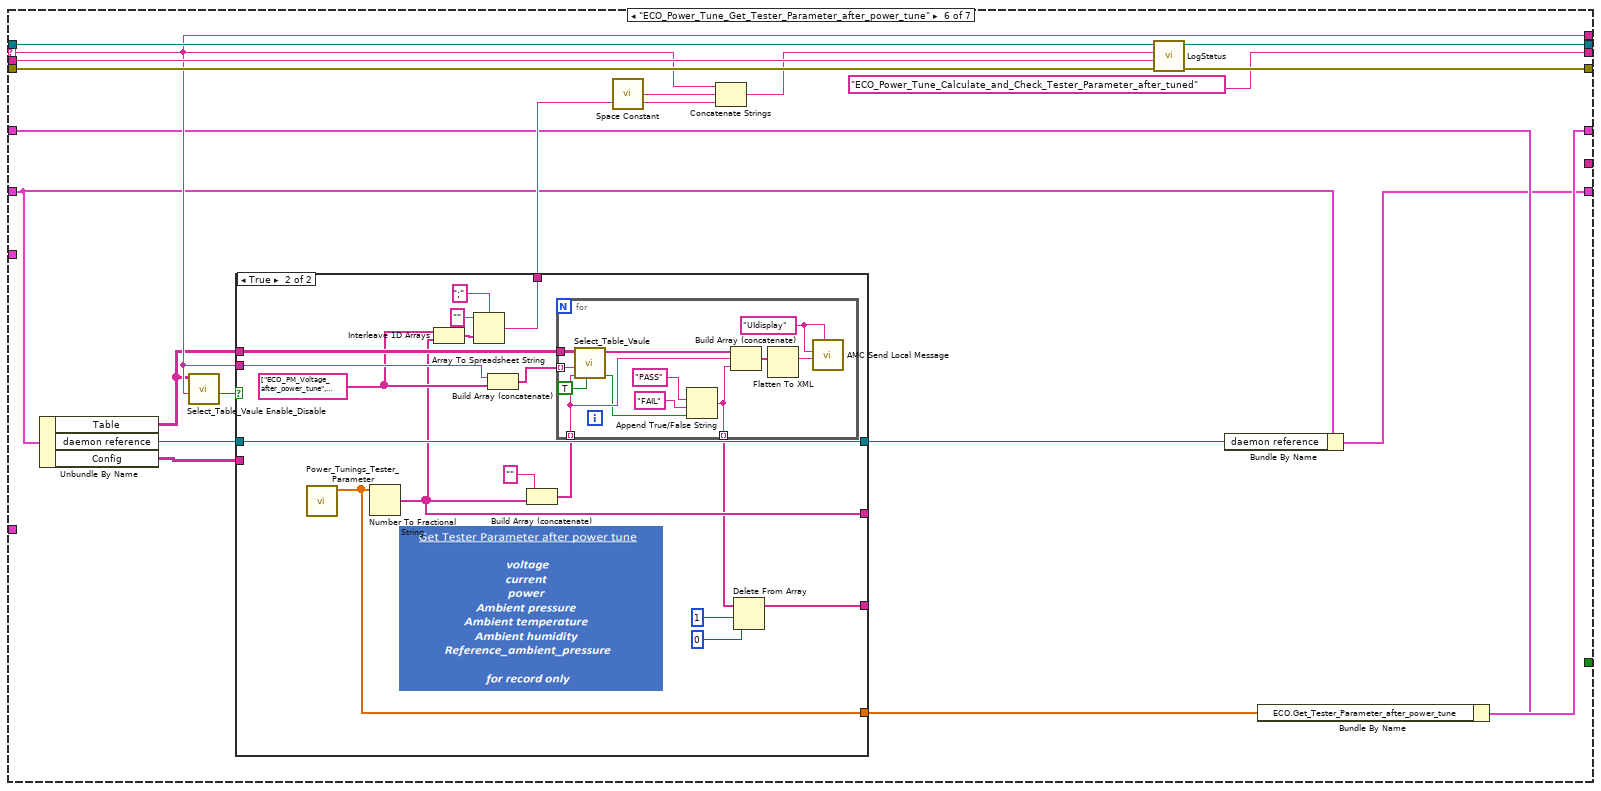
[diagram p12: hidden frame]
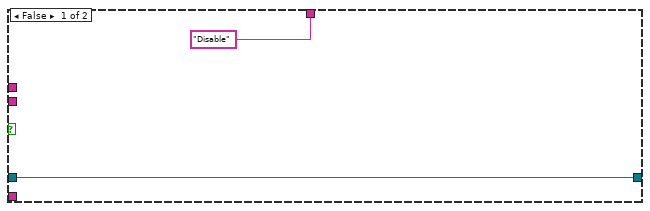
[diagram p13: hidden frame]
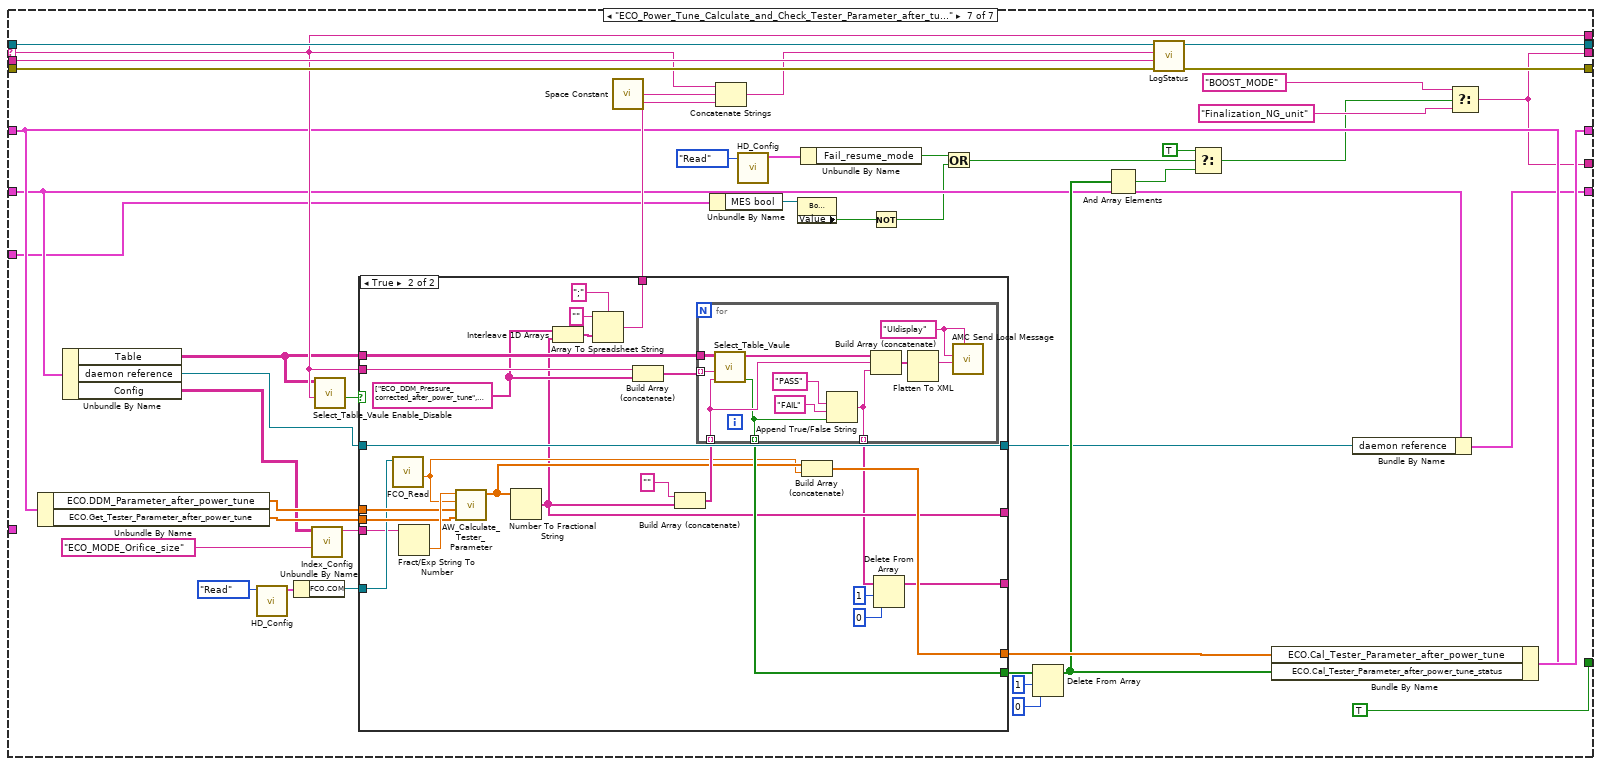
[diagram p14: hidden frame]
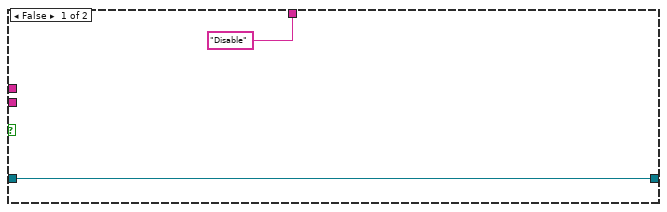
[diagram p15: hidden frame]
diagram:
  n1 = Flush Queue(queue="Message Queue out") -> (queue out=w4:T4)  [unwired: 1 in, 2 out]
  n2 = call "HD_Config.vi"("Step"=enum16{"Initial", "Write", "Read"}."Read") -> ("HD Config out"=w8:T5)  [unwired: 9 in, 1 out]
  n3 = call "AMC Send Local Message.vi"("error in (no error)"="error in (no error)", "Message Name"="ECO_Power_Tune_Set_Delta_Power_tune_value_to_DDM(A)", "Message Queue in"=w4) -> ("error out"=w13:errorcluster, "Message Queue out"=w14:T4)  [unwired: 7 in]
  n4 = while {
    tunnel: w14 -> [w47]
    tunnel: [w43] -> w6
    tunnel: w13 -> [w41]
    tunnel: [w38] -> w5
    shift-right: [w34] -> w10
    shift-left: "?" -> [w35]
    tunnel: w8 -> [w33]
    tunnel: [w29] -> w7
    shift-right: [w22] -> w1
    shift-left: "Data in" -> [w21]
    tunnel: "AllControls In" -> [w20]
    stop <- w23 stop-if-true
    n5 = Wait (ms)(milliseconds to wait=u32 1 ("等待时间（毫秒）")) -> ()  [unwired: 1 out]
    n6 = call "AMC Read Next Message.vi"("error in (no error)"=w41, "timeout (1ms)"=100, "Message Queue in"=w47) -> ("error out"=w40:errorcluster, "Message Value"=w31:string, "Message Name"=w45:string, "Message Queue out"=w46:T4)  [unwired: 1 in, 4 out]
    n7 = case shown="\"ECO_Power_Tune_Set_Delta_Power_tune_value_to_DDM(A)\"" w45 {
      selector: w45 -> [_ w72 w117 w155 w188 w261 w337]
      tunnel: w46 -> [w51 w80 w124 w161 w197 w270 w345]
      tunnel: [w51 w80 w124 w161 w197 w270 w345] -> w44
      tunnel: w40 -> [w50 _ _ w160 _ w269 w344]
      tunnel: [w50 w79 w123 w159 w196 w268 w343] -> w39
      tunnel: [_ w61 w111 _ w181 _ TRUE] -> w24
      tunnel: w35 -> [w49 w76 w107 w151 w193 w256 w335]
      tunnel: [w49 w57 w107 w151 w192 w265 w341] -> w34
      tunnel: w31 -> [_ w78 w122 w158 w195 w267 w342]
      tunnel: [_ w72 w117 w155 w188 w261 w337] -> w30
      tunnel: w33 -> [_ _ _ _ _ _ _]
      tunnel: [_ "ECO_Power_Tune_Motor_On_with_power_mode" "ECO_Power_Tune_Wait_for_X_sec_for_motor_speed_to_stabilise" "ECO_Power_Tune_Get_DDM_Parameter_after_power_tune" "ECO_Power_Tune_Get_Tester_Parameter_after_power_tune" "ECO_Power_Tune_Calculate_and_Check_Tester_Parameter_after_tuned" w331] -> w32
      tunnel: [_ w62 w112 _ w182 _ w331] -> w29
      tunnel: [w48 w52 w106 w148 w176 w252 w314] -> w22
      tunnel: w21 -> [w48 w55 w108 w148 w178 w254 w315]
      tunnel: w20 -> [_ _ _ _ _ _ w304]
      frame "假", Default {
      }
      frame "ECO_Power_Tune_Set_Delta_Power_tune_value_to_DDM(A)" {
        n8 = Unbundle By Name(w76) -> ("ECO.DDM_Parameter"=w70:dbl[], "ECO.Cal_Tester_Parameter"=w67:dbl[])
        n9 = Unbundle By Name(w55) -> ("Table"=w60:string[][], "daemon reference"=w59:refnum<k5>, "Config"=w58:string[][])
        n10 = Index Array(array=w70, index=2 ("索引")) -> (element=w66:dbl)
        n11 = Index Array(array=w67, index=1 ("索引")) -> (element=w65:dbl)
        n12 = Subtract(x=w66, y=w65) -> (x-y=w64:dbl)
        n13 = call "Select_Table_Vaule Enable_Disable.vi"("Action"=w72, "Table"=w60) -> ("Enable"=w71:bool)  [unwired: 8 in, 1 out]
        n14 = Multiply(x=w64, y=1000.0) -> (x*y=w54:dbl)
        n15 = case shown="True" w71 {
          tunnel: ["Disable" ("response") w87] -> w73
          tunnel: w60 -> [_ w97]
          tunnel: w72 -> [_ w96]
          tunnel: w59 -> [w83 w95]
          tunnel: w58 -> [_ w90]
          tunnel: w54 -> [_ w92]
          tunnel: [_ w89] -> w56
          tunnel: [_ w88] -> _
          tunnel: [_ w87] -> _
          tunnel: [_ w86] -> _
          tunnel: [w83 w85] -> w53
          frame False {
          }
          frame True {
            w103 = "UIdisplay" ("Process (\"\" - local)")
            n16 = To Long Integer(number=w92) -> (32bit integer=w93:i32)
            n17 = call "Index_Config.vi"("Action"="ECO_MODE_Drive_mode", "config"=w90) -> ("data"=w86:string)  [unwired: 9 in]
            n18 = call "set_aw_tune.vi"("Power Mode or Target Power in W"=w86, "Offset Power mW"=w93, "Index"=0, "daemon reference in"=w95) -> ("error out"=w89:errorcluster, "response"=w87:string, "daemon reference out"=w85:refnum<k5>)  [unwired: 4 in, 1 out]
            n19 = call "Select_Table_Vaule.vi"("Vaule"=w87, "Action"=w96, "Table"=w97) -> ("Result"=w98:bool, "vaule"=w104:string[])  [unwired: 7 in]
            n20 = Append True/False String(1:w98, 2:"FAIL" ("真字符串"), 3:"PASS" ("真字符串")) -> (0:w88:string)  [unwired: 1 in]
            n21 = Build Array (concatenate)(w104, w87, w88) -> (w102:string[])
            n22 = Flatten To XML(anything=w102) -> (xml string=w101:string)
            n23 = call "AMC Send Local Message.vi"("Process (\"\" - local)"=w103, "Message Value"=w101, "Message Name"=w103) -> ()  [unwired: 7 in, 2 out]
          }
        }
        n24 = call <vilib>:"Space Constant.vi"() -> ("String"=w74:string)
        n25 = Concatenate Strings(w72, w74, w73) -> (w75:string)
        n26 = Bundle By Name(cluster=w55, "daemon reference"=w53) -> (w52:T1)
        n27 = call "LogStatus.vi"("error in (no error)"=w56, "last message"=w78, "message"=w75) -> ("error  out"=w79:errorcluster)  [unwired: 8 in]
        n28 = Bundle By Name(cluster=w76, "ECO.Delta_P"=w54) -> (w57:T3)
        n29 = case shown="Error" w56 {
          tunnel: [_ TRUE] -> w61
          tunnel: [_ "Error"] -> w62
          frame No Error {
          }
          frame Error {
          }
        }
      }
      frame "ECO_Power_Tune_Motor_On_with_power_mode" {
        n30 = Unbundle By Name(w108) -> ("Table"=w116:string[][], "daemon reference"=w121:refnum<k5>, "Config"=w115:string[][])
        n31 = call "Select_Table_Vaule Enable_Disable.vi"("Action"=w117, "Table"=w116) -> ("Enable"=w118:bool)  [unwired: 8 in, 1 out]
        n32 = case shown="True" w118 {
          tunnel: w121 -> [w128 w146]
          tunnel: [TRUE w136] -> _
          tunnel: [w128 w140] -> w105
          tunnel: ["Disable" ("response") w132] -> w109
          tunnel: w117 -> [_ w139]
          tunnel: w116 -> [_ w138]
          tunnel: w115 -> [_ w134]
          tunnel: "ECO_MODE_Drive_mode" -> [_ w135]
          tunnel: [_ w133] -> w110
          tunnel: [_ w132] -> _
          tunnel: [_ w131] -> _
          tunnel: [_ w130] -> _
          frame False {
          }
          frame True {
            (unwired) "ECO" ("Power Mode")
            w145 = "UIdisplay" ("Process (\"\" - local)")
            n33 = call "Index_Config.vi"("Action"=w135, "config"=w134) -> ("data"=w130:string)  [unwired: 9 in]
            n34 = call "drive_motor.vi"("Power Mode"=w130, "daemon reference in"=w146) -> ("error out"=w133:errorcluster, "response"=w132:string, "daemon reference out"=w140:refnum<k5>)  [unwired: 6 in, 1 out]
            n35 = call "Select_Table_Vaule.vi"("Vaule"=w132, "Action"=w139, "Table"=w138) -> ("Result"=w136:bool, "vaule"=w137:string[])  [unwired: 7 in]
            n36 = Append True/False String(1:w136, 2:"FAIL" ("真字符串"), 3:"PASS" ("真字符串")) -> (0:w131:string)  [unwired: 1 in]
            n37 = Build Array (concatenate)(w137, w132, w131) -> (w144:string[])
            n38 = Flatten To XML(anything=w144) -> (xml string=w143:string)
            n39 = call "AMC Send Local Message.vi"("Process (\"\" - local)"=w145, "Message Value"=w143, "Message Name"=w145) -> ()  [unwired: 7 in, 2 out]
          }
        }
        n40 = call <vilib>:"Space Constant.vi"() -> ("String"=w120:string)
        n41 = Concatenate Strings(w117, w120, w109) -> (w119:string)
        n42 = Bundle By Name(cluster=w108, "daemon reference"=w105) -> (w106:T1)
        n43 = call "LogStatus.vi"("error in (no error)"=w110, "last message"=w122, "message"=w119) -> ("error  out"=w123:errorcluster)  [unwired: 8 in]
        n44 = case shown="Error" w110 {
          tunnel: [_ TRUE] -> w111
          tunnel: [_ "Error"] -> w112
          frame No Error {
          }
          frame Error {
          }
        }
      }
      frame "ECO_Power_Tune_Wait_for_X_sec_for_motor_speed_to_stabilise" {
        # "来之Config"
        n45 = Unbundle By Name(w148) -> ("Config"=w153:string[][])
        n46 = call "Index_Config.vi"("Action"="ECO_MODE_Stabilisation_time", "config"=w153) -> ("data"=w147:string)  [unwired: 9 in]
        n47 = Get Date/Time In Seconds() -> (seconds since 1Jan1904=w150:timestamp)
        n48 = Search and Replace String(input string=w155, search string="X" ("搜索字符串")) -> (result string=w154:string)  [unwired: 6 in, 3 out]
        n49 = Fract/Exp String To Number(string=w147) -> (number=w149:dbl)  [unwired: 3 in, 1 out]
        n50 = while {
          tunnel: w150 -> [w168]
          tunnel: w149 -> [w165]
          tunnel: [w164] -> _
          stop <- w164 stop-if-true
          n51 = Get Date/Time In Seconds() -> (seconds since 1Jan1904=w169:timestamp)
          n52 = Subtract(x=w169, y=w168) -> (x-y=w167:dbl)
          n53 = call "6-AlarmStatus.vi"("Step"=enum16{"Initial", "Write", "Read"}."Read") -> ("AlarmValue Out"=w172:bool[])  [unwired: 9 in, 1 out]
          n54 = Greater Or Equal?(x=w167, y=w165) -> (x >= y?=w166:bool)
          n55 = call "Stop.vi"("Step"=enum16{"Initial", "Write", "Read"}."Read") -> ("Stop Out"=w170:bool)  [unwired: 9 in, 1 out]
          n56 = call "Exit.vi"("Step"=enum16{"Initial", "Write", "Read"}."Read" ("step")) -> ("Exit Out"=w174:bool)  [unwired: 9 in, 1 out]
          n57 = Or Array Elements(Boolean array=w172) -> (logical OR=w171:bool)
          n58 = Compound Arithmetic op=OR(w166, w170, w174, w171) -> (w164:bool)
          n59 = Wait (ms)(milliseconds to wait=u32 1 ("等待时间（毫秒）")) -> ()  [unwired: 1 out]
        }
        n60 = call "LogStatus.vi"("error in (no error)"=w160, "last message"=w158, "message"=w154) -> ("error  out"=w159:errorcluster)  [unwired: 8 in]
      }
      frame "ECO_Power_Tune_Get_DDM_Parameter_after_power_tune" {
        n61 = Unbundle By Name(w178) -> ("Table"=w187:string[][], "daemon reference"=w194:refnum<k5>, "Config"=w185:string[][])
        n62 = call "Select_Table_Vaule Enable_Disable.vi"("Action"=w188, "Table"=w187) -> ("Enable"=w186:bool)  [unwired: 8 in, 1 out]
        n63 = case shown="True" w186 {
          tunnel: w194 -> [w201 w226]
          tunnel: [w201 w225] -> w177
          tunnel: ["Disable" ("software string") w220] -> w189
          tunnel: w188 -> [_ w223]
          tunnel: w187 -> [_ w227]
          tunnel: w185 -> [_ _]
          tunnel: [_ w214] -> w183
          tunnel: [_ w217] -> w179
          tunnel: T6[] ["voltage", "current", "power", "speed", "measured_power", "pressure", "lsi_magnet_temp", "fisf_magnet_temp", "iir_magnet_temp"] ("Parameter") -> [_ w211]
          tunnel: [_ w206] -> _
          tunnel: [_ w202] -> _
          frame False {
          }
          frame True {
            w212 = string[] ["ECO_DDM_Voltage_after_power_tune", "ECO_DDM_Current_after_power_tune", "ECO_DDM_Power_after_power_tune", "ECO_DDM_Speed_after_power_tune", "ECO_DDM_Measured_Power_after_power_tune", "ECO_DDM_Pressure_after_power_tune", "ECO_lsi_magnet_temp_after_power_tune", "ECO_fisf_magnet_temp_after_power_tune", "ECO_iir_magnet_temp_after_power_tune"]
            n64 = for {
              tunnel: [w233] -> w210 mode=indexing
              tunnel: [w232] -> w217
              tunnel: [w229] -> w213 mode=indexing
              tunnel: w211 -> [w230] mode=indexing
              shift-right: [w234] -> w225
              shift-left: w226 -> [w235]
              n65 = Build Array(w230) -> (w228:T6[])
              n66 = call "get_parameter.vi"("Parameter"=w228, "daemon reference in"=w235) -> ("error out"=w232:errorcluster, "response"=w233:string, "values"=w231:dbl[], "daemon reference out"=w234:refnum<k5>)  [unwired: 5 in, 1 out]
              n67 = Index Array(array=w231) -> (element=w229:dbl)  [unwired: 1 in]
            }
            n68 = in-place {
              w240 = 1000.0
              n69 = in-place-array #1(w213, 3, 5) -> (w239:dbl, w236:dbl)
              n70 = Divide(x=w239, y=w240) -> (x/y=w238:dbl)
              n71 = Divide(x=w236, y=w240) -> (x/y=w237:dbl)
              n72 = in-place-array #1(w238, w237) -> (w214:dbl[])  [unwired: 2 out]
            }
            n73 = Array To Spreadsheet String(delimiter (Tab)=",", array=w210, 3:"" ("format string")) -> (spreadsheet string=w209:string)
            n74 = Number To Fractional String(number=w214) -> (F-format string=w206:string[])  [unwired: 3 in]
            n75 = Interleave 1D Arrays(w212, w206) -> (w221:string[])
            n76 = Build Array (concatenate)(w223, w212) -> (w224:string[])
            n77 = Array To Spreadsheet String(delimiter (Tab)=";" ("分隔符(Tab)"), array=w221, 3:"" ("格式字符串")) -> (spreadsheet string=w220:string)
            n78 = Build Array (concatenate)(w209, w206) -> (w222:string[])
            n79 = for {
              tunnel: w227 -> [w246]
              tunnel: w222 -> [w244] mode=indexing
              tunnel: w224 -> [w243] mode=indexing
              tunnel: [w241] -> w203 mode=indexing
              w251 = "UIdisplay" ("Process (\"\" - local)")
              n80 = call "Select_Table_Vaule.vi"("Vaule"=w244, "Action"=w243, "Table"=w246) -> ("Result"=w242:bool, "vaule"=w245:string[])  [unwired: 7 in]
              n81 = Append True/False String(1:w242, 2:"FAIL" ("真字符串"), 3:"PASS" ("真字符串")) -> (0:w241:string)  [unwired: 1 in]
              n82 = Build Array (concatenate)(w245, w244, w241) -> (w250:string[])
              n83 = Flatten To XML(anything=w250) -> (xml string=w249:string)
              n84 = call "AMC Send Local Message.vi"("Process (\"\" - local)"=w251, "Message Value"=w249, "Message Name"=w251) -> ()  [unwired: 7 in, 2 out]
            }
            n85 = Delete From Array(array=w203, length=1 ("长度"), index=0 ("索引")) -> (array with subset deleted=w202:string[])  [unwired: 1 out]
          }
        }
        n86 = call <vilib>:"Space Constant.vi"() -> ("String"=w191:string)
        n87 = Concatenate Strings(w188, w191, w189) -> (w190:string)
        n88 = Bundle By Name(cluster=w193, "ECO.DDM_Parameter_after_power_tune"=w183) -> (w192:T3)
        n89 = call "LogStatus.vi"("error in (no error)"=w179, "last message"=w195, "message"=w190) -> ("error  out"=w196:errorcluster)  [unwired: 8 in]
        n90 = Bundle By Name(cluster=w178, "daemon reference"=w177) -> (w176:T1)
        n91 = case shown="Error" w179 {
          tunnel: [_ TRUE] -> w181
          tunnel: [_ "Error"] -> w182
          frame No Error {
          }
          frame Error {
          }
        }
      }
      frame "ECO_Power_Tune_Get_Tester_Parameter_after_power_tune" {
        n92 = Unbundle By Name(w254) -> ("Table"=w260:string[][], "daemon reference"=w266:refnum<k5>, "Config"=w258:string[][])
        n93 = call "Select_Table_Vaule Enable_Disable.vi"("Action"=w261, "Table"=w260) -> ("Enable"=w259:bool)  [unwired: 8 in, 1 out]
        n94 = case shown="True" w259 {
          tunnel: w266 -> [w272 w288]
          tunnel: [w272 w288] -> w253
          tunnel: ["Disable" ("software string") w280] -> w262
          tunnel: w261 -> [_ w286]
          tunnel: w260 -> [_ w289]
          tunnel: w258 -> [_ _]
          tunnel: [_ w279] -> w257
          tunnel: [_ w277] -> _
          tunnel: [_ w273] -> _
          frame False {
          }
          frame True {
            w278 = string[] ["ECO_PM_Voltage_after_power_tune", "ECO_PM_Current_after_power_tune", "ECO_PM_Power_after_power_tune", "ECO_Ambient_Pressure_after_power_tune", "ECO_Ambient_Temperature_after_power_tune", "ECO_Ambient_humidity_after_power_tune", "ECO_Tester_Reference_Ambient_Pressure_after_power_tune"]
            n95 = call "Power_Tunings_Tester_Parameter.vi"() -> ("Power_Tuning_Tester_Parameter"=w279:dbl[])  [unwired: 11 in]
            n96 = Number To Fractional String(number=w279) -> (F-format string=w277:string[])  [unwired: 3 in]
            n97 = Interleave 1D Arrays(w278, w277) -> (w283:string[])
            n98 = Array To Spreadsheet String(delimiter (Tab)=";" ("分隔符(Tab)"), array=w283, 3:"" ("格式字符串")) -> (spreadsheet string=w280:string)
            n99 = Build Array (concatenate)(w286, w278) -> (w287:string[])
            n100 = Build Array (concatenate)("", w277) -> (w285:string[])
            n101 = for {
              tunnel: w289 -> [w296]
              tunnel: w285 -> [w294] mode=indexing
              tunnel: w287 -> [w293] mode=indexing
              tunnel: [w290] -> w274 mode=indexing
              w301 = "UIdisplay" ("Process (\"\" - local)")
              n102 = call "Select_Table_Vaule.vi"("Boolean"=TRUE, "Vaule"=w294, "Action"=w293, "Table"=w296) -> ("Result"=w292:bool, "vaule"=w295:string[])  [unwired: 6 in]
              n103 = Append True/False String(1:w292, 2:"FAIL" ("真字符串"), 3:"PASS" ("真字符串")) -> (0:w290:string)  [unwired: 1 in]
              n104 = Build Array (concatenate)(w295, w294, w290) -> (w300:string[])
              n105 = Flatten To XML(anything=w300) -> (xml string=w299:string)
              n106 = call "AMC Send Local Message.vi"("Process (\"\" - local)"=w301, "Message Value"=w299, "Message Name"=w301) -> ()  [unwired: 7 in, 2 out]
            }
            n107 = Delete From Array(array=w274, length=1 ("长度"), index=0 ("索引")) -> (array with subset deleted=w273:string[])  [unwired: 1 out]
          }
        }
        n108 = call <vilib>:"Space Constant.vi"() -> ("String"=w264:string)
        n109 = Concatenate Strings(w261, w264, w262) -> (w263:string)
        n110 = call "LogStatus.vi"("error in (no error)"=w269, "last message"=w267, "message"=w263) -> ("error  out"=w268:errorcluster)  [unwired: 8 in]
        n111 = Bundle By Name(cluster=w254, "daemon reference"=w253) -> (w252:T1)
        n112 = Bundle By Name(cluster=w256, "ECO.Get_Tester_Parameter_after_power_tune"=w257) -> (w265:T3)
      }
      frame "ECO_Power_Tune_Calculate_and_Check_Tester_Parameter_after_tuned" {
        n113 = Unbundle By Name(w335) -> ("ECO.DDM_Parameter_after_power_tune"=w322:dbl[], "ECO.Get_Tester_Parameter_after_power_tune"=w321:dbl[])
        n114 = Unbundle By Name(w315) -> ("Table"=w318:string[][], "daemon reference"=w317:refnum<k5>, "Config"=w316:string[][])
        n115 = call "HD_Config.vi"("Step"=enum16{"Initial", "Write", "Read"}."Read") -> ("HD Config out"=w323:T5)  [unwired: 9 in, 1 out]
        n116 = Unbundle By Name(w323) -> ("FCO.COM"=w320:refnum<visa-resource-name>)
        n117 = call "Index_Config.vi"("Action"="ECO_MODE_Orifice_size", "config"=w316) -> ("data"=w319:string)  [unwired: 9 in]
        n118 = call "Select_Table_Vaule Enable_Disable.vi"("Action"=w337, "Table"=w318) -> ("Enable"=w336:bool)  [unwired: 8 in, 1 out]
        n119 = case shown="True" w336 {
          tunnel: w317 -> [w347 w371]
          tunnel: [w347 w371] -> w313
          tunnel: ["Disable" ("software string") w362] -> w338
          tunnel: w337 -> [_ w369]
          tunnel: w318 -> [_ w372]
          tunnel: [_ w354] -> w330
          tunnel: [_ w370] -> w329
          tunnel: w322 -> [_ w359]
          tunnel: w321 -> [_ w358]
          tunnel: w320 -> [_ w357]
          tunnel: w319 -> [_ w356]
          tunnel: [_ w352] -> _
          tunnel: [_ w348] -> _
          frame False {
          }
          frame True {
            w355 = string[] ["ECO_DDM_Pressure_corrected_after_power_tune", "ECO_DDM_Real_Power_after_power_tune", "ECO_Delta_V_after_power_tune", "ECO_Flow_rate_after_power_tune", "ECO_AW_after_power_tune"]
            n120 = call "FCO_Read.vi"("VISA in"=w357) -> ("Pressure(Pa)"=w353:dbl)  [unwired: 7 in, 3 out]
            n121 = Fract/Exp String To Number(string=w356) -> (number=w361:dbl)  [unwired: 3 in, 1 out]
            n122 = call "AW_Calculate_Tester_Parameter.vi"("Tester Parameter"=w358, "DDM Parameter"=w359, "AW_Box_Pressure/Stag Total-Static Pressure rise"=w353, "Orifice_Plate_Diameter"=w361) -> ("Calculate Tester Parameter"=w360:dbl[])  [unwired: 7 in]
            n123 = Number To Fractional String(number=w360) -> (F-format string=w352:string[])  [unwired: 3 in]
            n124 = Interleave 1D Arrays(w355, w352) -> (w365:string[])
            n125 = Array To Spreadsheet String(delimiter (Tab)=";" ("分隔符(Tab)"), array=w365, 3:"" ("格式字符串")) -> (spreadsheet string=w362:string)
            n126 = Build Array (concatenate)(w369, w355) -> (w368:string[])
            n127 = Build Array (concatenate)("", w352) -> (w367:string[])
            n128 = for {
              tunnel: w372 -> [w378]
              tunnel: w367 -> [w376] mode=indexing
              tunnel: w368 -> [w375] mode=indexing
              tunnel: [w374] -> w370 mode=indexing
              tunnel: [w373] -> w349 mode=indexing
              w383 = "UIdisplay" ("Process (\"\" - local)")
              n129 = call "Select_Table_Vaule.vi"("Vaule"=w376, "Action"=w375, "Table"=w378) -> ("Result"=w374:bool, "vaule"=w377:string[])  [unwired: 7 in]
              n130 = Append True/False String(1:w374, 2:"FAIL" ("真字符串"), 3:"PASS" ("真字符串")) -> (0:w373:string)  [unwired: 1 in]
              n131 = Build Array (concatenate)(w377, w376, w373) -> (w382:string[])
              n132 = Flatten To XML(anything=w382) -> (xml string=w381:string)
              n133 = call "AMC Send Local Message.vi"("Process (\"\" - local)"=w383, "Message Value"=w381, "Message Name"=w383) -> ()  [unwired: 7 in, 2 out]
            }
            n134 = Build Array (concatenate)(w360, w353) -> (w354:dbl[])
            n135 = Delete From Array(array=w349, length=1 ("长度"), index=0 ("索引")) -> (array with subset deleted=w348:string[])  [unwired: 1 out]
          }
        }
        n136 = call <vilib>:"Space Constant.vi"() -> ("String"=w340:string)
        n137 = Unbundle By Name(w304) -> ("MES bool"=w308:refnum<vi>)
        n138 = Concatenate Strings(w337, w340, w338) -> (w339:string)
        n139 = call "HD_Config.vi"("Step"=enum16{"Initial", "Write", "Read"}."Read") -> ("HD Config out"=w307:T5)  [unwired: 9 in, 1 out]
        n140 = property class="Bool (严格)"(reference=w308) -> ("Value"=w310:bool)  [unwired: 1 in, 2 out]
        n141 = Unbundle By Name(w307) -> ("Fail_resume_mode"=w309:bool)
        n142 = Not(x=w310) -> (.not. x?=w312:bool)
        n143 = Or(x=w309, y=w312) -> (x .or. y?=w311:bool)
        n144 = Delete From Array(array=w329, length=1 ("长度"), index=0 ("索引")) -> (array with subset deleted=w326:bool[])  [unwired: 1 out]
        n145 = And Array Elements(Boolean array=w326) -> (logical AND=w303:bool)
        n146 = call "LogStatus.vi"("error in (no error)"=w344, "last message"=w342, "message"=w339) -> ("error  out"=w343:errorcluster)  [unwired: 8 in]
        n147 = Select(t=TRUE, s=w311, f=w303) -> (s? t:f=w302:bool)
        n148 = Bundle By Name(cluster=w335, "ECO.Cal_Tester_Parameter_after_power_tune"=w330, "ECO.Cal_Tester_Parameter_after_power_tune_status"=w326) -> (w341:T3)
        n149 = Bundle By Name(cluster=w315, "daemon reference"=w313) -> (w314:T1)
        n150 = Select(t="BOOST_MODE", s=w302, f="Finalization_NG_unit") -> (s? t:f=w331:string)
      }
    }
    n151 = call "6-AlarmStatus.vi"("Step"=enum16{"Initial", "Write", "Read"}."Read") -> ("AlarmValue Out"=w18:bool[])  [unwired: 9 in, 1 out]
    n152 = call "Stop.vi"("Step"=enum16{"Initial", "Write", "Read"}."Read") -> ("Stop Out"=w26:bool)  [unwired: 9 in, 1 out]
    n153 = call "Exit.vi"("Step"=enum16{"Initial", "Write", "Read"}."Read" ("step")) -> ("Exit Out"=w25:bool)  [unwired: 9 in, 1 out]
    n154 = Or Array Elements(Boolean array=w18) -> (logical OR=w17:bool)
    n155 = Compound Arithmetic op=OR(w24, w26, w25, w17) -> (w23:bool)
    n156 = call "AMC Run Step.vi"("Message Queue In"=w44, "Message Name"=w32, "Message Value"=w30, "error in (no error)"=w39, "Mli/Sig"=FALSE) -> ("Message Queue Out"=w43:T4, "error out"=w38:errorcluster)  [unwired: 13 in]
  }
  "Message Queue Out" <- w6
  "error out" <- w5
  "Data" <- w10
  "Flow" <- w7
  "Data out" <- w1
